vi "Might be useful.vi"   [LabVIEW 2021]
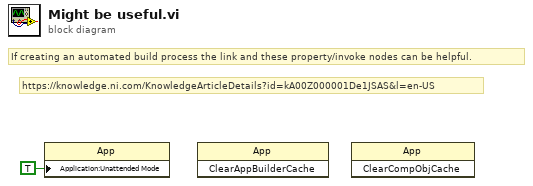
[diagram p0: block diagram]
diagram:
  # "If creating an automated build process the link and these property/invoke nodes can be helpful."
  # "https://knowledge.ni.com/KnowledgeArticleDetails?id=kA00Z000001De1JSAS&l=en-US"
  n1 = property class="App"("Application:Unattended Mode"=TRUE) -> ()  [unwired: 2 in, 2 out]
  n2 = invoke class="App" method="ClearAppBuilderCache"() -> ()  [unwired: 3 in, 3 out]
  n3 = invoke class="App" method="ClearCompObjCache"() -> ()  [unwired: 3 in, 3 out]
